vi "Init Plugin.vi"(8 "error in (no error)":errorcluster, 10 "Plugin":string, 11 "Execution UI in":refnum<class "Execution UI.lvclass">) -> (0 "error out":errorcluster, 3 "Execution UI out":refnum<class "Execution UI.lvclass">)   [LabVIEW 2020, in "Execution UI.lvclass"]
uses:
  Execution UI.lvclass
  Execution UI.lvclass/Execution UI.ctl
  Plugin Loader/Plugin Loader.lvclass
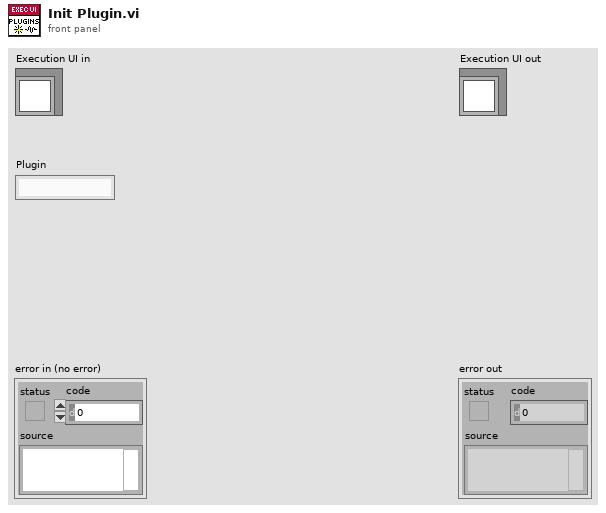
[diagram p1: front panel]
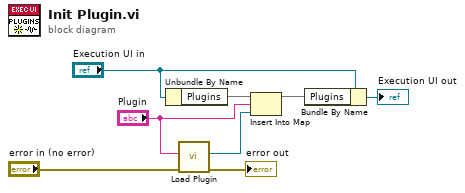
[diagram p0: block diagram]
diagram:
  n1 = Unbundle By Name("Execution UI in") -> ("Plugins"=w4:map{string, refnum<class "Plugin.lvclass">})
  n2 = call "Load Plugin.vi"("error in (no error)"="error in (no error)", "Plugin"="Plugin") -> ("error out"=→"error out":errorcluster, "Plugin"=w1:refnum<class "Plugin.lvclass">)  [unwired: 8 in]
  n3 = Insert Into Map(map in=w4, key="Plugin", value=w1) -> (map out=w2:map{string, refnum<class "Plugin.lvclass">})  [unwired: 2 out]
  n4 = Bundle By Name(cluster="Execution UI in", "Plugins"=w2) -> (→"Execution UI out":refnum<class "Execution UI.lvclass">)
